vi "Set FP state.vi"(11 "Laser State":T2) -> (0 "Laser Power":T1(ring)=enum."Disabled and Grayed Out", 1 "stop laser":T1(ring), 2 "warm laser":T1(ring), 3 "Fire laser":T1(ring))   [LabVIEW 2022 SP3, in "Laser View.lvclass"]
uses:
  Laser View.lvclass
  Laser State Data/Laser State.ctl
  Laser View.lvclass/Laser View.ctl
  Laser State Data/Laser State Data.lvclass
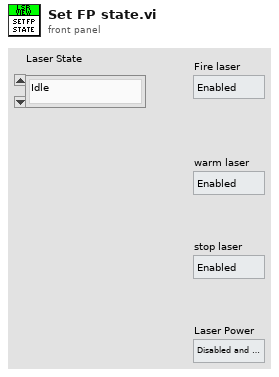
[diagram p1: front panel]
types:
  T1 = enum8{"Enabled", "Disabled", "Disabled and Grayed Out"}
  T2 = typedef "Laser State Data.lvclass/Laser State.ctl" = enum16{"Idle", "Warming", "Ready", "Firing"}
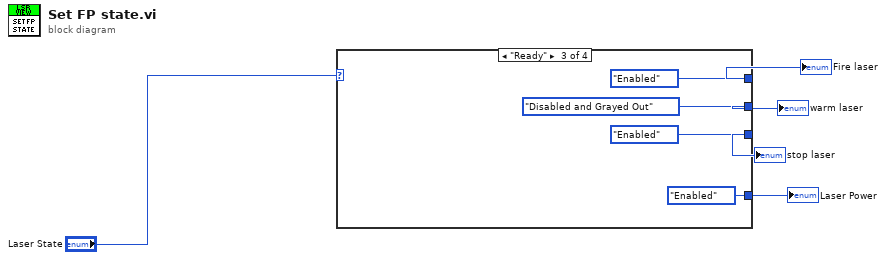
[diagram p0: block diagram]
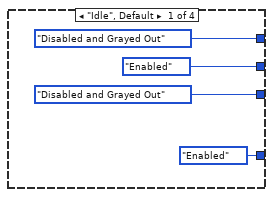
[diagram p2: hidden frame]
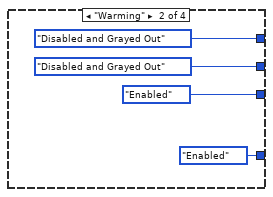
[diagram p3: hidden frame]
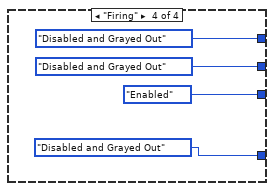
[diagram p4: hidden frame]
diagram:
  n1 = case shown="\"Ready\"" "Laser State" {
    tunnel: [T1."Enabled" ("Disabled") T1."Disabled and Grayed Out" ("Disabled") T1."Disabled and Grayed Out" ("Disabled") T1."Disabled and Grayed Out" ("Disabled")] -> w3
    tunnel: [T1."Disabled and Grayed Out" ("Disabled") T1."Enabled" ("Disabled") T1."Enabled" ("Disabled") T1."Enabled" ("Disabled")] -> w4
    tunnel: [T1."Disabled and Grayed Out" ("Disabled") T1."Disabled and Grayed Out" ("Disabled") T1."Enabled" ("Disabled") T1."Disabled and Grayed Out" ("Disabled")] -> w5
    tunnel: [T1."Enabled" ("Disabled") T1."Enabled" ("Disabled") T1."Enabled" ("Disabled") T1."Disabled and Grayed Out" ("Disabled")] -> w1
    frame "Idle", Default {
    }
    frame "Warming" {
    }
    frame "Ready" {
    }
    frame "Firing" {
    }
  }
  "Fire laser" <- w5
  "stop laser" <- w4
  "warm laser" <- w3
  "Laser Power" <- w1
